vi "Check Health.vi"(8 "error in":errorcluster, 11 "System Session":refnum<k21>="localhost") -> (0 "error out":errorcluster, 1 "FIFO":T1)   [LabVIEW 2024]
uses:
  Type Definitions/FIFO_Health.ctl
  Type Definitions/CPU_and_memory.ctl
  <resource>/objmgr/nisysapi.rc
  <vilib>/NI_Real-Time Target Support.lvlib
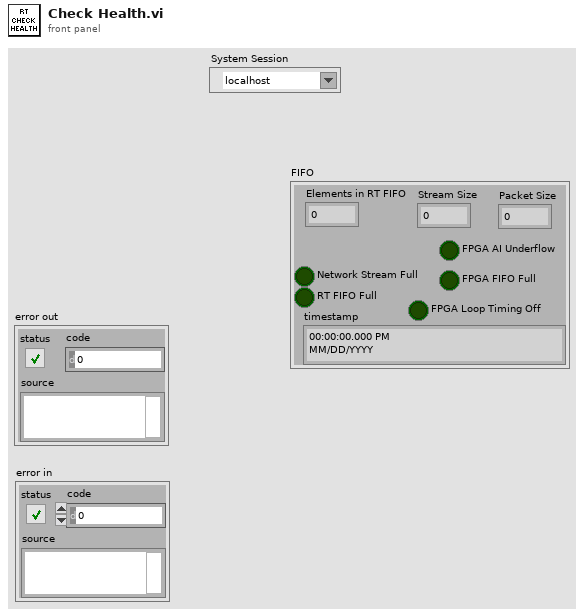
[diagram p1: front panel]
types:
  T1 = typedef "FIFO_Health.ctl" = cluster{"Elements in RT FIFO":i32, "Network Stream Full":bool, "RT FIFO Full":bool, "FPGA AI Underflow":bool, "FPGA FIFO Full":bool, "FPGA Loop Timing Off":bool, "timestamp":timestamp, "Stream Size":u32, "Packet Size":u32}
  T2 = typedef "CPU_and_memory.ctl" = cluster{"CPU 1 (%)":dbl, "CPU 2 (%)":dbl, "Free Virtual\nMemory(%)":dbl, "Free Hard drive space (%)":dbl, "Free Physical\n Memory (%)":dbl}
  T3 = typedef "NI_Real-Time Target Support.lvlib/RT CPU Load.ctl" = cluster{"Total (%)":dbl, "Time Critical (%)":dbl, "Timed Structures (%)":dbl, "High (%)":dbl, "Above Normal (%)":dbl, "Normal (%)":dbl, "Background (%)":dbl, "Idle (%)":dbl, "ISR (%)":dbl}
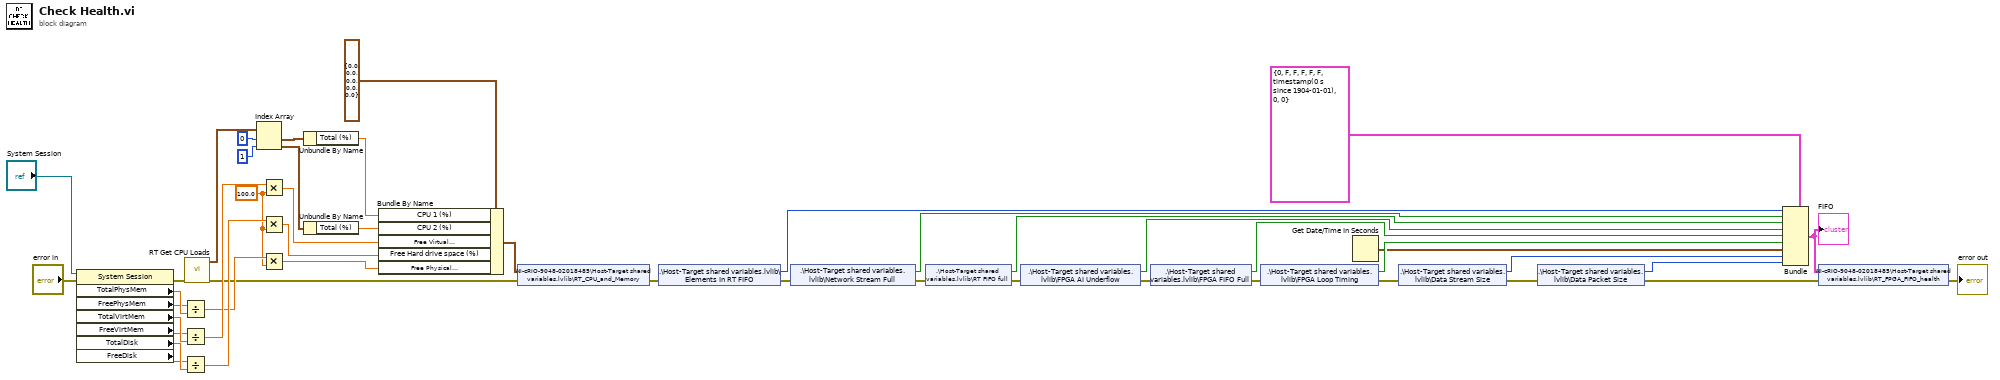
[diagram p0: block diagram]
diagram:
  w2 = 100.0 ("y")
  n1 = property class="System Session"(reference="System Session", error in="error in") -> (error out=w29:errorcluster, "TotalPhysMem"=w33:dbl, "FreePhysMem"=w32:dbl, "TotalVirtMem"=w37:dbl, "FreeVirtMem"=w36:dbl, "TotalDisk"=w40:dbl, "FreeDisk"=w39:dbl)  [unwired: 1 out]
  n2 = Divide(x=w32, y=w33) -> (x/y=w34:dbl)
  n3 = Divide(x=w36, y=w37) -> (x/y=w35:dbl)
  n4 = Divide(x=w39, y=w40) -> (x/y=w38:dbl)
  n5 = call <vilib>:"RT Get CPU Loads.vi"("error in (no error)"=w29) -> ("error out"=w31:errorcluster, "CPU loads"=w43:T3[])  [unwired: 9 in]
  n6 = Index Array(array=w43, index #1=0 ("index"), index #2=1 ("index")) -> (element #1=w42:T3, element #2=w41:T3)
  n7 = Multiply(x=w35, y=w2) -> (x*y=w26:dbl)
  n8 = Multiply(x=w38, y=w2) -> (x*y=w27:dbl)
  n9 = Multiply(x=w34, y=w2) -> (x*y=w25:dbl)
  n10 = Unbundle By Name(w42) -> ("Total (%)"=w24:dbl)
  n11 = Unbundle By Name(w41) -> ("Total (%)"=w23:dbl)
  n12 = Bundle By Name(cluster=T2 {"CPU 1 (%)"=0.0, "CPU 2 (%)"=0.0, "Free Virtual\nMemory(%)"=0.0, "Free Hard drive space (%)"=0.0, "Free Physical\n Memory (%)"=0.0} ("RT_CPU_and_Memory"), "CPU 1 (%)"=w24, "CPU 2 (%)"=w23, "Free Virtual\nMemory(%)"=w26, "Free Hard drive space (%)"=w27, "Free Physical\n Memory (%)"=w25) -> (w22:T2)
  n13 = shared-variable "NI-cRIO-9048-02018485\\Host-Target shared variables.lvlib\\RT_CPU_and_Memory"(w22, error in=w31) -> (error out=w30:errorcluster)
  n14 = shared-variable ".\\Host-Target shared variables.lvlib\\Elements In RT FIFO"(error in=w30) -> (w19:i32, error out=w18:errorcluster)
  n15 = shared-variable ".\\Host-Target shared variables.lvlib\\Network Stream Full"(error in=w18) -> (w20:bool, error out=w17:errorcluster)
  n16 = shared-variable ".\\Host-Target shared variables.lvlib\\RT FIFO full"(error in=w17) -> (w21:bool, error out=w16:errorcluster)
  n17 = shared-variable ".\\Host-Target shared variables.lvlib\\FPGA AI Underflow"(error in=w16) -> (w13:bool, error out=w15:errorcluster)
  n18 = shared-variable ".\\Host-Target shared variables.lvlib\\FPGA FIFO Full"(error in=w15) -> (w12:bool, error out=w14:errorcluster)
  n19 = shared-variable ".\\Host-Target shared variables.lvlib\\FPGA Loop Timing"(error in=w14) -> (w11:bool, error out=w7:errorcluster)
  n20 = Get Date/Time In Seconds() -> (seconds since 1Jan1904=w10:timestamp)
  n21 = shared-variable ".\\Host-Target shared variables.lvlib\\Data Stream Size"(error in=w7) -> (w6:u32, error out=w5:errorcluster)
  n22 = shared-variable ".\\Host-Target shared variables.lvlib\\Data Packet Size"(error in=w5) -> (w3:u32, error out=w4:errorcluster)
  n23 = Bundle(cluster=T1 {"Elements in RT FIFO"=0, "Network Stream Full"=FALSE, "RT FIFO Full"=FALSE, "FPGA AI Underflow"=FALSE, "FPGA FIFO Full"=FALSE, "FPGA Loop Timing Off"=FALSE, "timestamp"=timestamp(0 s since 1904-01-01), "Stream Size"=0, "Packet Size"=0} ("FIFO 2"), "Elements in RT FIFO"=w19, "Network Stream Full"=w20, "RT FIFO Full"=w21, "FPGA AI Underflow"=w13, "FPGA FIFO Full"=w12, "FPGA Loop Timing Off"=w11, "timestamp"=w10, "Stream Size"=w6, "Packet Size"=w3) -> (w8:T1)
  "FIFO" <- w8
  n24 = shared-variable "NI-cRIO-9048-02018485\\Host-Target shared variables.lvlib\\RT_FPGA_FIFO_health"(w8, error in=w4) -> (error out=→"error out":errorcluster)
